vi "coordinate.vi"(1 "Cluster":cluster{"Horizontal":i32, "Vertical":i32}) -> (0 "output cluster":T1)   [LabVIEW 2014]
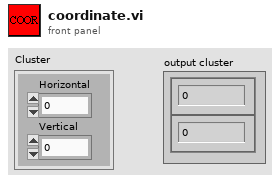
[diagram p1: front panel]
types:
  T1 = cluster{"Numeric Control":dbl, "Numeric Control":dbl}
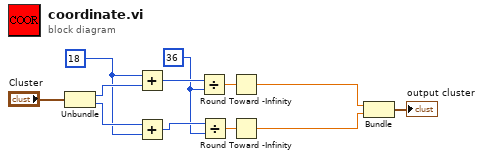
[diagram p0: block diagram]
diagram:
  w6 = 36
  w9 = 18
  n1 = Unbundle("Cluster") -> ("Horizontal"=w11:i32, "Vertical"=w10:i32)
  n2 = Add(x=w9, y=w11) -> (x+y=w8:i32)
  n3 = Add(x=w10, y=w9) -> (x+y=w7:i32)
  n4 = Divide(x=w8, y=w6) -> (x/y=w5:dbl)
  n5 = Divide(x=w7, y=w6) -> (x/y=w4:dbl)
  n6 = Round Toward -Infinity(1:w5) -> (0:w2:dbl)
  n7 = Round Toward -Infinity(1:w4) -> (0:w1:dbl)
  n8 = Bundle(w2, w1) -> (→"output cluster":cluster{dbl, dbl})  [unwired: 1 in]
